vi "Quiver Constructor.vi"(0 "3D Quiver Datatype.lvclass in":refnum<class "3D Quiver Datatype.lvclass">, 1 "Nx Matrix":sgl[][](array[numeric]), 2 "Ny Matrix":sgl[][](array[numeric]), 3 "Nz matrix":sgl[][](array[numeric]), 5 "x vector":sgl[][](array[numeric]), 7 "y vector":sgl[][](array[numeric]), 9 "z matrix":sgl[][](array[numeric]), 11 "error in (no error)":errorcluster, 14 "Plot ID":i32) -> (4 "3D Quiver Datatype.lvclass out":refnum<class "3D Quiver Datatype.lvclass">, 15 "error out":errorcluster)   [LabVIEW 2017, in "3D Quiver Datatype.lvclass"]
uses:
  <vilib>/Math Plots/3D Math Plots/3D Quiver/3D Quiver Datatype/3D Quiver Datatype.lvclass
  <vilib>/Math Plots/3D Math Plots/3D Quiver/3D Quiver Datatype/3D Quiver Datatype.lvclass/3D Quiver Datatype.ctl
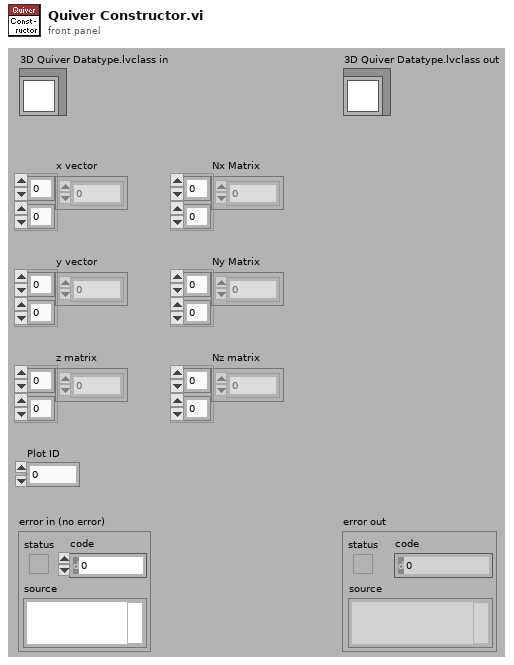
[diagram p1: front panel]
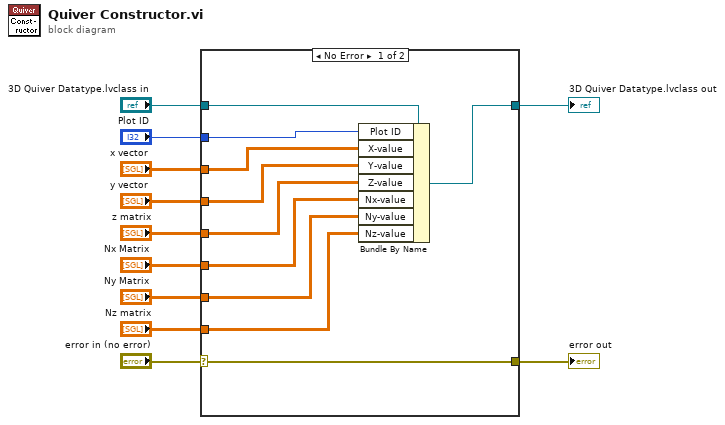
[diagram p0: block diagram]
diagram:
  n1 = case shown="No Error" "error in (no error)" {
    selector: "error in (no error)" -> [w16 w23]
    tunnel: "Plot ID" -> [w12 _]
    tunnel: [w16 w23] -> w10
    tunnel: "x vector" -> [w21 _]
    tunnel: "y vector" -> [w20 _]
    tunnel: "z matrix" -> [w19 _]
    tunnel: "3D Quiver Datatype.lvclass in" -> [w18 w22]
    tunnel: [w17 w22] -> w4
    tunnel: "Nx Matrix" -> [w15 _]
    tunnel: "Ny Matrix" -> [w14 _]
    tunnel: "Nz matrix" -> [w13 _]
    frame No Error {
      n2 = Bundle By Name(cluster=w18, "Plot ID"=w12, "X-value"=w21, "Y-value"=w20, "Z-value"=w19, "Nx-value"=w15, "Ny-value"=w14, "Nz-value"=w13) -> (w17:refnum<class "3D Quiver Datatype.lvclass">)
    }
    frame Error {
    }
  }
  "error out" <- w10
  "3D Quiver Datatype.lvclass out" <- w4
